vi "ReversedEngineering GetDepNodeIndex.vi"(1 "classInfo":T1, 2 "classInfoArray":T1[](array[typedef]), 3 "AllNodes":refnum<class "AbstractNode.lvclass">[](array[class]), 5 "error in (no error)":errorcluster) -> (11 "depNodes":i32[](array[numeric]), 13 "noOfAgg":i32[](array[numeric]), 15 "inheritanceNode":i32, 16 "compAggNodes":i32[](array[numeric]), 17 "noOfCompAgg":i32[](array[numeric]), 18 "aggNodes":i32[](array[numeric]), 19 "error out":errorcluster)   [LabVIEW 2020]
uses:
  <resource>/Framework/Providers/Open_GDS/UML/ReversedEngineering/ReversedEngineering ClassInfoType.ctl
  <resource>/Framework/Providers/Open_GDS/UML/UMLEditor/UMLEditor_VisibilityType.ctl
  <resource>/Framework/Providers/Open_GDS/UML/ReversedEngineering/ReversedEngineering AttributeInfoType.ctl
  <resource>/Framework/Providers/Open_GDS/ClassProviders/Common/CommonVIs/CommonVIs_AttributeDataType.ctl
  <resource>/Framework/Providers/Open_GDS/UML/ReversedEngineering/ReversedEngineering_ClassDependencyDetailsType.ctl
  <resource>/Framework/Providers/Open_GDS/ClassProviders/Common/ScriptingFunctions/SubVIs/Scripting_ViDependencyType.ctl
  <resource>/Framework/Providers/Open_GDS/UML/AbstractNode_class/AbstractNode.lvclass
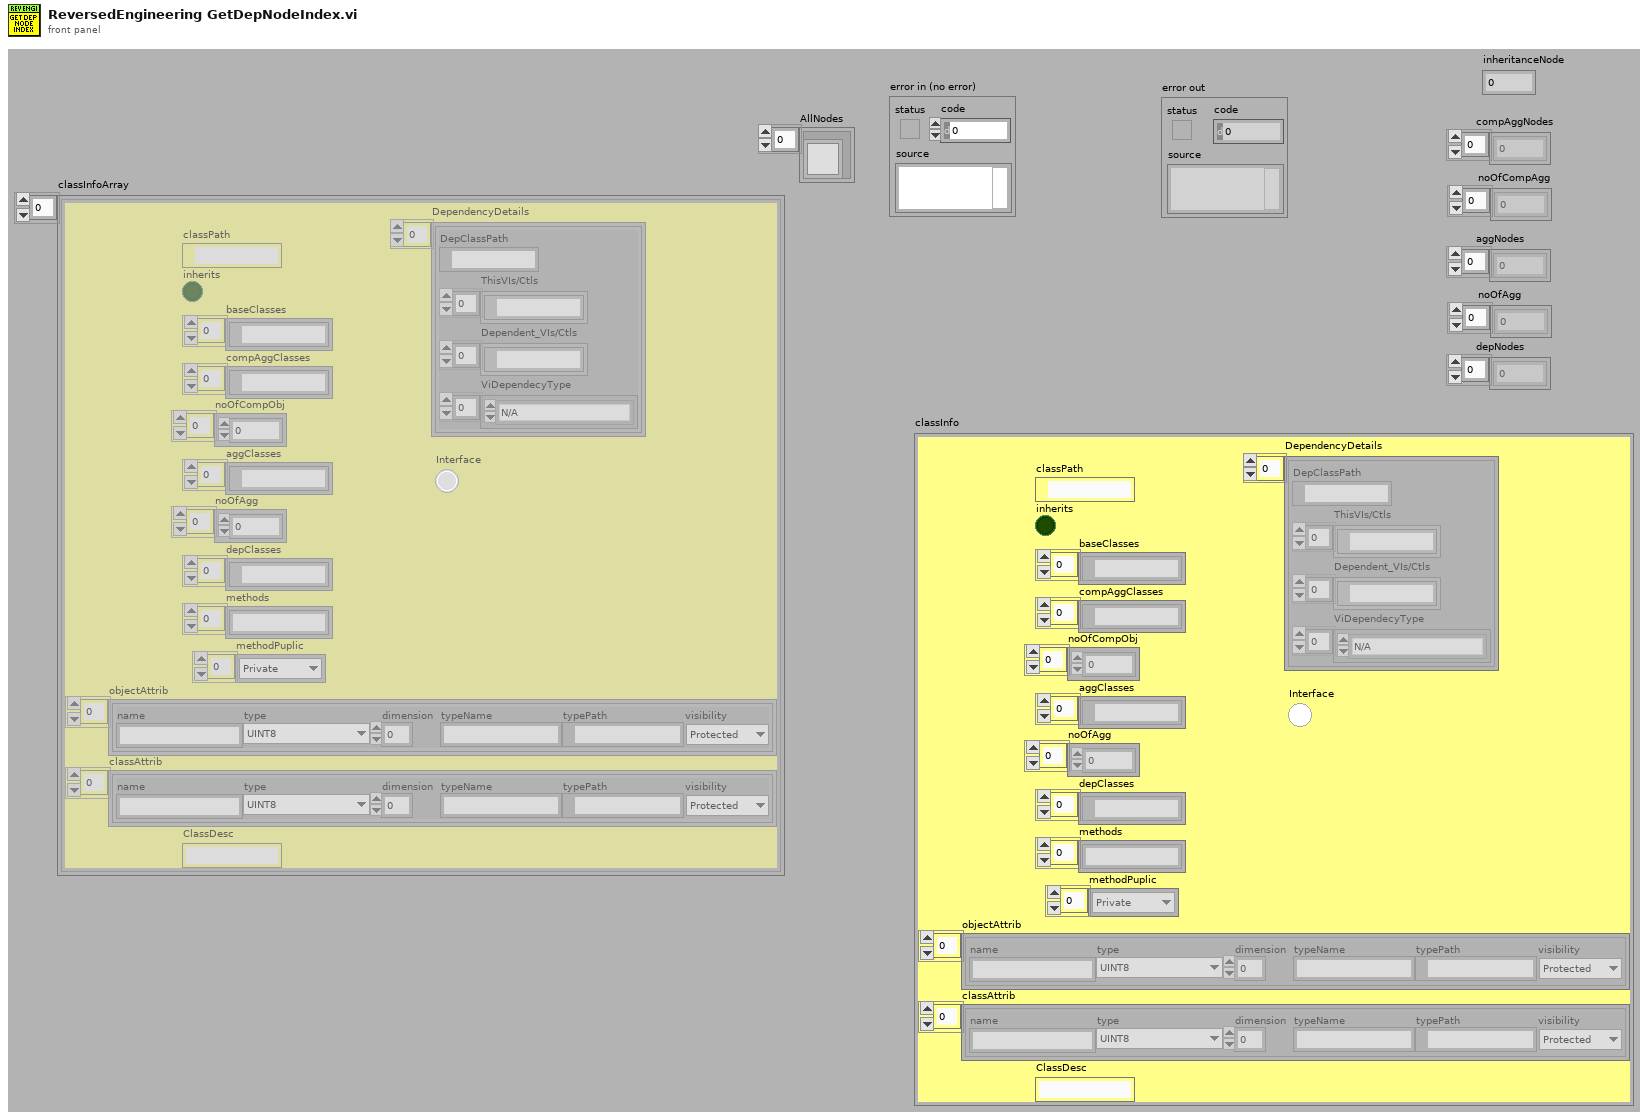
[diagram p1: front panel]
types:
  T1 = typedef "ReversedEngineering ClassInfoType.ctl" = cluster{"classPath":path, "inherits":bool, "baseClasses":path[], "compAggClasses":path[], "noOfCompObj":i32[], "aggClasses":path[], "noOfAgg":i32[], "depClasses":path[], "methods":string[], "methodPuplic":T2[], "objectAttrib":T3[], "classAttrib":T3[], "ClassDesc":string, "DependencyDetails":T5[], "Interface":bool}
  T2 = typedef "UMLEditor_VisibilityType.ctl" = enum16{"Public", "Private", "Protected"}
  T3 = typedef "ReversedEngineering AttributeInfoType.ctl" = cluster{"name":string, "type":T4, "dimension":i32, "typeName":string, "typePath":path, "visibility":T2}
  T4 = typedef "CommonVIs_AttributeDataType.ctl" = enum16{"UINT8", "INT8", "UINT16", "INT16", "UINT32", "INT32", "UINT64", "INT64", "SGL", "DBL", "EXT", "CSG", "CDB", "CXT", "TimeStamp", "STRING", "PATH", "BOOL", "ENUM", "RefNum", "VIRefNum", "LabVIEW Class", "Cluster", "Variant", "TypeDef", "Waveform", "LabVIEW Object", "Other", "void"}
  T5 = typedef "ReversedEngineering_ClassDependencyDetailsType.ctl" = cluster{"DepClassPath":path, "ThisVIs/Ctls":path[], "Dependent_VIs/Ctls":path[], "ViDependecyType":T6[]}
  T6 = typedef "Scripting_ViDependencyType.ctl" = enum16{"N/A", "Launches"}
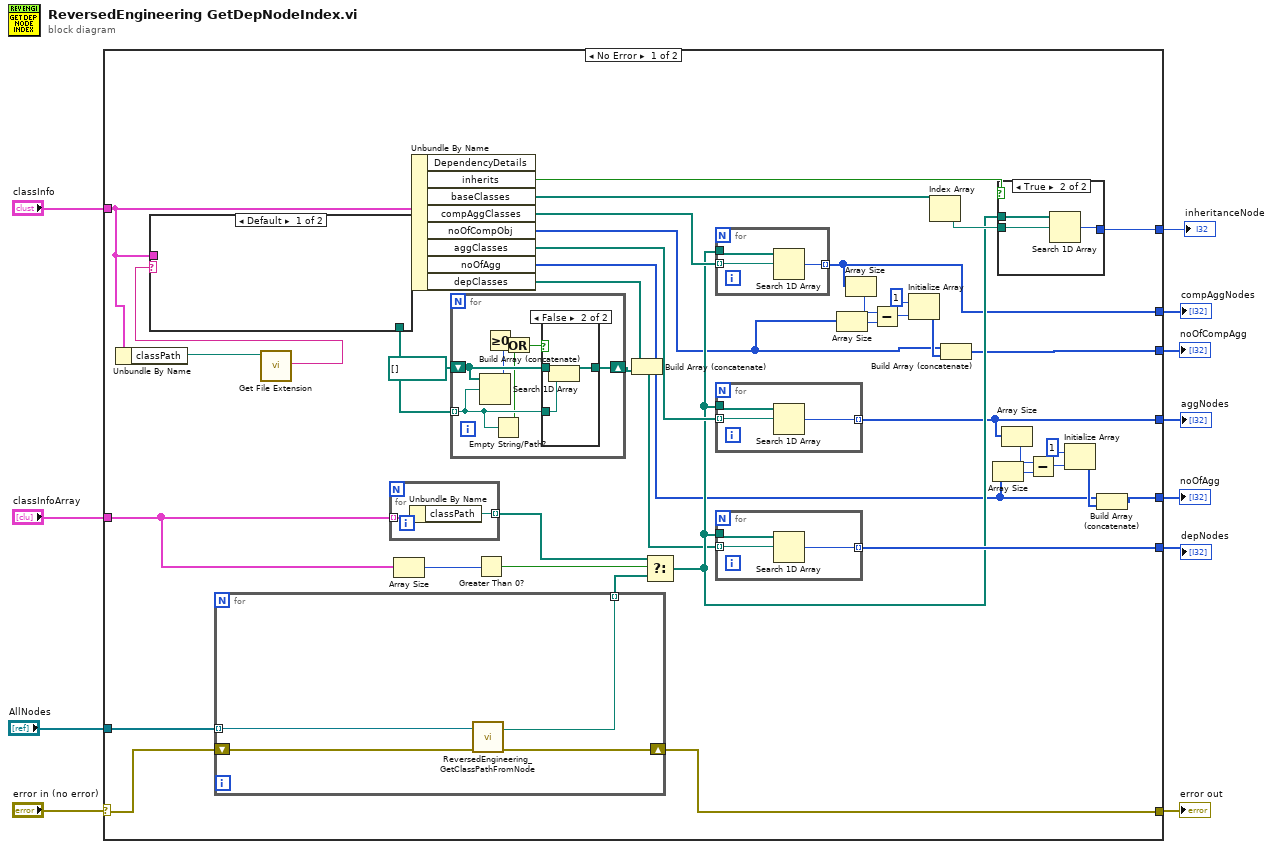
[diagram p0: block diagram]
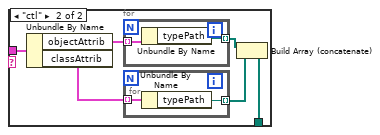
[diagram p2: hidden frame]
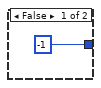
[diagram p4: hidden frame]
diagram:
  n1 = case shown="No Error" "error in (no error)" {
    selector: "error in (no error)" -> [w38 w92]
    tunnel: [w37 w92] -> w11
    tunnel: "classInfo" -> [w30 _]
    tunnel: "classInfoArray" -> [w44 _]
    tunnel: [w49 _] -> w7
    tunnel: [w27 _] -> w6
    tunnel: [w23 _] -> w5
    tunnel: [w14 _] -> w4
    tunnel: [w13 _] -> w3
    tunnel: [w45 _] -> w2
    tunnel: "AllNodes" -> [w39 _]
    frame No Error {
      n2 = Unbundle By Name(w30) -> ("classPath"=w29:path)
      n3 = for {
        tunnel: w39 -> [w76] mode=indexing
        shift-right: [w74] -> w37
        shift-left: w38 -> [w75]
        tunnel: [w73] -> w36 mode=indexing
        n4 = call <resource>:"ReversedEngineering_GetClassPathFromNode.vi"("reference"=w76, "error IO"=w75) -> ("Path"=w73:path, "error out"=w74:errorcluster)  [unwired: 2 in, 14 out]
      }
      n5 = call <vilib>:"Get File Extension.vi"("file"=w29) -> ("lowercase file extension"=w28:string)  [unwired: 1 in, 9 out]
      n6 = case shown="Default" w28 {
        tunnel: [_ w53] -> w35
        tunnel: w30 -> [_ w52]
        frame Default {
        }
        frame "ctl" {
          n7 = Unbundle By Name(w52) -> ("objectAttrib"=w57:T3[], "classAttrib"=w56:T3[])
          n8 = for {
            tunnel: w57 -> [w61] mode=indexing
            tunnel: [w60] -> w55 mode=indexing
            n9 = Unbundle By Name(w61) -> ("typePath"=w60:path)
          }
          n10 = for {
            tunnel: w56 -> [w59] mode=indexing
            tunnel: [w58] -> w54 mode=indexing
            n11 = Unbundle By Name(w59) -> ("typePath"=w58:path)
          }
          n12 = Build Array (concatenate)(w55, w54) -> (w53:path[])
        }
      }
      n13 = for {
        tunnel: w44 -> [w91] mode=indexing
        tunnel: [w90] -> w40 mode=indexing
        n14 = Unbundle By Name(w91) -> ("classPath"=w90:path)
      }
      n15 = Array Size(array=w44) -> (size(s)=w43:i32)
      n16 = Unbundle By Name(w30) -> ("inherits"=w50:bool, "baseClasses"=w51:path[], "compAggClasses"=w47:path[], "noOfCompObj"=w20:i32[], "aggClasses"=w46:path[], "noOfAgg"=w12:i32[], "depClasses"=w33:path[])  [unwired: 1 out]
      n17 = for {
        tunnel: w35 -> [w65] mode=indexing
        shift-right: [w68] -> w32
        shift-left: path[] [] -> [w67]
        n18 = Search 1D Array(1D array=w67, element=w65) -> (index of element=w66:i32)  [unwired: 1 out]
        n19 = Greater Or Equal To 0?(x=w66) -> (x >= 0?=w64:bool)
        n20 = Empty String/Path?(string/path=w65) -> (empty?=w63:bool)
        n21 = Or(x=w64, y=w63) -> (x .or. y?=w62:bool)
        n22 = case shown="False" w62 {
          tunnel: w65 -> [_ w72]
          tunnel: [w69 w70] -> w68
          tunnel: w67 -> [w69 w71]
          frame True {
          }
          frame False {
            n23 = Build Array (concatenate)(w71, w72) -> (w70:path[])
          }
        }
      }
      n24 = Greater Than 0?(x=w43) -> (x > 0?=w42:bool)
      n25 = Build Array (concatenate)(w33, w32) -> (w31:path[])
      n26 = Select(t=w40, s=w42, f=w36) -> (s? t:f=w41:path[])
      n27 = for {
        tunnel: w47 -> [w84] mode=indexing
        tunnel: w41 -> [w85]
        tunnel: [w83] -> w27 mode=indexing
        n28 = Search 1D Array(1D array=w85, element=w84) -> (index of element=w83:i32)  [unwired: 1 out]
      }
      n29 = for {
        tunnel: w46 -> [w81] mode=indexing
        tunnel: w41 -> [w82]
        tunnel: [w80] -> w14 mode=indexing
        n30 = Search 1D Array(1D array=w82, element=w81) -> (index of element=w80:i32)  [unwired: 1 out]
      }
      n31 = for {
        tunnel: w31 -> [w78] mode=indexing
        tunnel: w41 -> [w79]
        tunnel: [w77] -> w45 mode=indexing
        n32 = Search 1D Array(1D array=w79, element=w78) -> (index of element=w77:i32)  [unwired: 1 out]
      }
      n33 = Array Size(array=w20) -> (size(s)=w25:i32)
      n34 = Array Size(array=w27) -> (size(s)=w26:i32)
      n35 = Subtract(x=w26, y=w25) -> (x-y=w24:i32)
      n36 = Initialize Array(1 ("Numeric"), w24) -> (w22:i32[])
      n37 = Index Array(array=w51) -> (element=w48:path)  [unwired: 1 in]
      n38 = Build Array (concatenate)(w20, w22) -> (w23:i32[])
      n39 = Array Size(array=w12) -> (size(s)=w16:i32)
      n40 = case shown="True" w50 {
        tunnel: [-1 ("inheritanceNode") w87] -> w49
        tunnel: w41 -> [_ w89]
        tunnel: w48 -> [_ w88]
        frame False {
        }
        frame True {
          n41 = Search 1D Array(1D array=w89, element=w88) -> (index of element=w87:i32)  [unwired: 1 out]
        }
      }
      n42 = Array Size(array=w14) -> (size(s)=w15:i32)
      n43 = Subtract(x=w15, y=w16) -> (x-y=w17:i32)
      n44 = Initialize Array(1 ("Numeric"), w17) -> (w18:i32[])
      n45 = Build Array (concatenate)(w12, w18) -> (w13:i32[])
    }
    frame Error {
    }
  }
  "error out" <- w11
  "compAggNodes" <- w6
  "inheritanceNode" <- w7
  "noOfCompAgg" <- w5
  "noOfAgg" <- w3
  "aggNodes" <- w4
  "depNodes" <- w2
